vi "FileWrite.vi"(5 "DataArray":dbl[](array[numeric]), 7 "Time Stamp":timestamp, 8 "Error In":errorcluster, 9 "FileFormat":string[](array[string]), 10 "Index":i32, 11 "refnum in":refnum<file>) -> (0 "Error Out":errorcluster, 3 "Byte Stream File Refnum":refnum<file>)   [LabVIEW 2017]
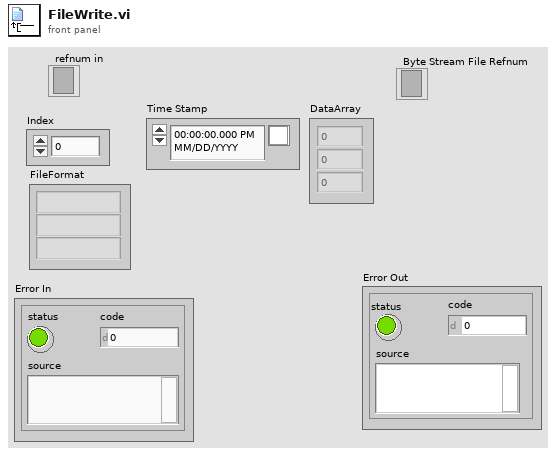
[diagram p1: front panel]
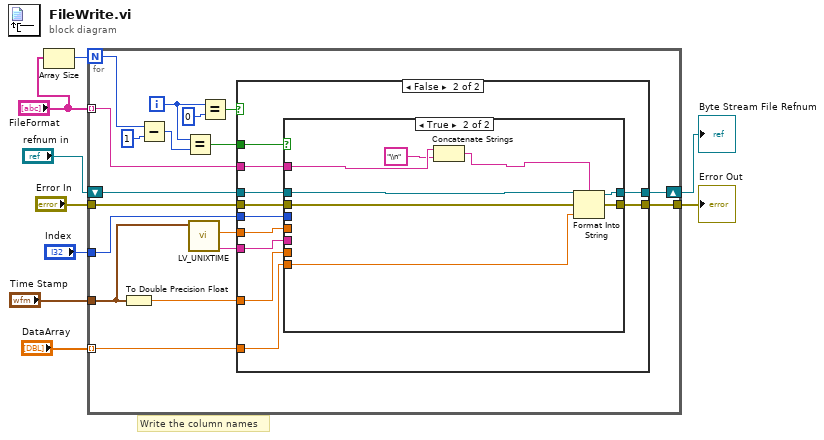
[diagram p0: block diagram]
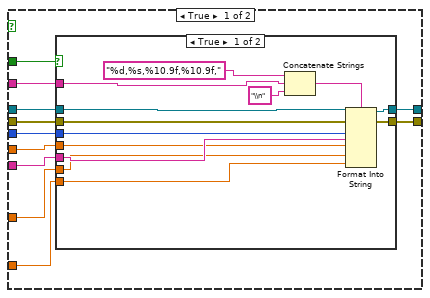
[diagram p2: hidden frame]
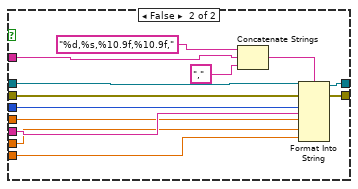
[diagram p3: hidden frame]
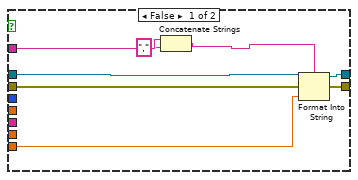
[diagram p4: hidden frame]
diagram:
  # "Write the column names"
  n1 = Array Size(array="FileFormat") -> (size(s)=w9:i32)
  n2 = for {
    N: w9 -> [w20]
    tunnel: [w23] -> w7
    tunnel: "Error In" -> [w21]
    shift-right: [w22] -> w8
    shift-left: "refnum in" -> [w17]
    tunnel: "Time Stamp" -> [w11]
    tunnel: "Index" -> [w16]
    tunnel: "DataArray" -> [w13] mode=indexing
    tunnel: "FileFormat" -> [w12] mode=indexing
    i -> [w25]
    n3 = To Double Precision Float(number=w11) -> (double precision float=w10:dbl)
    n4 = Subtract(x=w20, y=1 ("x")) -> (x-y=w19:i32)
    n5 = Equal?(x=w25, y=w19) -> (x = y?=w24:bool)
    n6 = call "LV_UNIXTIME.vi"("current time"=w11) -> ("date/time string"=w15:string, "UNIX time (s)"=w14:dbl)  [unwired: 9 in]
    n7 = Equal?(x=w25, y=0) -> (x = y?=w26:bool)
    n8 = case shown="False" w26 {
      tunnel: w17 -> [w38 w75]
      tunnel: w24 -> [w37 w74]
      tunnel: [w35 w72] -> w23
      tunnel: [w36 w73] -> w22
      tunnel: w21 -> [w34 w71]
      tunnel: w16 -> [w33 w70]
      tunnel: w15 -> [w32 w69]
      tunnel: w14 -> [w31 w68]
      tunnel: w13 -> [w30 w67]
      tunnel: w12 -> [w29 w66]
      tunnel: w10 -> [w28 w65]
      frame True {
        n9 = case shown="True" w37 {
          tunnel: w38 -> [w51 w64]
          tunnel: [w50 w63] -> w36
          tunnel: [w49 w62] -> w35
          tunnel: w34 -> [w48 w61]
          tunnel: w33 -> [w46 w59]
          tunnel: w32 -> [w45 w58]
          tunnel: w31 -> [w44 w57]
          tunnel: w30 -> [w43 w56]
          tunnel: w29 -> [w41 w54]
          tunnel: w28 -> [w39 w53]
          frame True {
            n10 = Concatenate Strings("%d,%s,%10.9f,%10.9f," ("format string"), w41, "\\n" ("string")) -> (w42:string)
            n11 = Format Into String(format string=w42, initial string=w51, error in=w48, w46, w45, w44, w39, w43) -> (resulting string=w50:refnum<file>, error out=w49:errorcluster)
          }
          frame False {
            n12 = Concatenate Strings("%d,%s,%10.9f,%10.9f," ("format string"), w54, "," ("string")) -> (w55:string)
            n13 = Format Into String(format string=w55, initial string=w64, error in=w61, w59, w58, w57, w53, w56) -> (resulting string=w63:refnum<file>, error out=w62:errorcluster)
          }
        }
      }
      frame False {
        n14 = case shown="True" w74 {
          tunnel: w75 -> [w83 w91]
          tunnel: [w82 w90] -> w73
          tunnel: [w81 w89] -> w72
          tunnel: w71 -> [w80 w88]
          tunnel: w70 -> [_ _]
          tunnel: w69 -> [_ _]
          tunnel: w68 -> [_ _]
          tunnel: w67 -> [w79 w87]
          tunnel: w66 -> [w78 w86]
          tunnel: w65 -> [_ _]
          frame False {
            n15 = Concatenate Strings(w78, "," ("string")) -> (w76:string)
            n16 = Format Into String(format string=w76, initial string=w83, error in=w80, w79) -> (resulting string=w82:refnum<file>, error out=w81:errorcluster)
          }
          frame True {
            n17 = Concatenate Strings(w86, "\\n" ("string")) -> (w85:string)
            n18 = Format Into String(format string=w85, initial string=w91, error in=w88, w87) -> (resulting string=w90:refnum<file>, error out=w89:errorcluster)
          }
        }
      }
    }
  }
  "Byte Stream File Refnum" <- w8
  "Error Out" <- w7
